vi "TDT-Wait For Inactive Tag.vi"(0 "RPcoX in":refnum<k7>, 9 "Timeout (ms)":dbl=2000.0, 11 "error in (no error)":errorcluster) -> (4 "RPcoX out":refnum<k7>, 15 "error out":errorcluster)   [LabVIEW 2020]
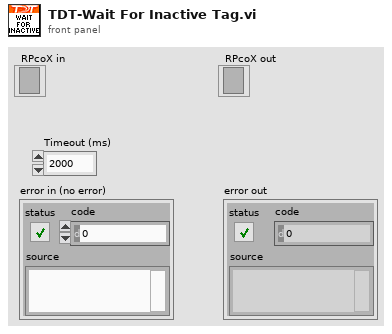
[diagram p1: front panel]
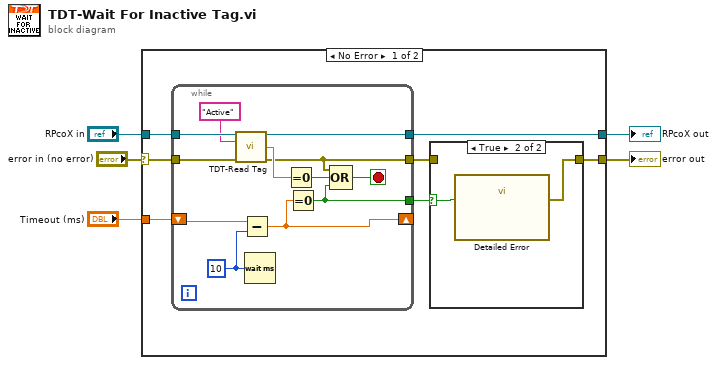
[diagram p0: block diagram]
diagram:
  n1 = case shown="No Error" "error in (no error)" {
    selector: "error in (no error)" -> [w9 w28]
    tunnel: "RPcoX in" -> [w12 w29]
    tunnel: [w11 w29] -> w4
    tunnel: [w6 w28] -> w5
    tunnel: "Timeout (ms)" -> [w10 _]
    frame No Error {
      n2 = while {
        tunnel: w12 -> [w27]
        tunnel: w9 -> [w26]
        tunnel: [w25] -> w11
        tunnel: [w18] -> w7
        shift-right: [w16] -> _
        shift-left: w10 -> [w22]
        tunnel: [w17] -> w8
        stop <- w19 stop-if-true
        w21 = u32 10 ("milliseconds to wait")
        n3 = call "TDT-Read Tag.vi"("RPcox"=w27, "Name"="Active", "error in"=w26) -> ("RPcox Out"=w25:refnum<k7>, "GetTagVal"=w23:sgl, "error out"=w18:errorcluster)  [unwired: 10 in]
        n4 = Subtract(x=w22, y=w21) -> (x-y=w16:dbl)
        n5 = Wait (ms)(milliseconds to wait=w21) -> ()  [unwired: 1 out]
        n6 = Equal To 0?(x=w23) -> (x = 0?=w20:bool)
        n7 = Equal To 0?(x=w16) -> (x = 0?=w17:bool)
        n8 = Compound Arithmetic op=OR(w18, w20, w17) -> (w19:bool)
      }
      n9 = case shown="True" w8 {
        selector: w8 -> [_ w15]
        tunnel: w7 -> [w13 _]
        tunnel: [w13 w14] -> w6
        frame False {
        }
        frame True {
          n10 = call "Detailed Error"("Error?"=w15) -> ("detailed error"=w14:errorcluster)  [unwired: 14 in]
        }
      }
    }
    frame Error {
    }
  }
  "error out" <- w5
  "RPcoX out" <- w4
